vi "Mask Joysticks.vi"(6 "Operator POVs":i16[](array[numeric]), 7 "Driver Axes":dbl[](array[numeric])=[6.0, 0.0, 0.0, 1.0], 8 "Operator Buttons":bool[](array[boolean])=[FALSE, FALSE, FALSE, FALSE, FALSE, FALSE, FALSE, FALSE, FALSE, FALSE], 9 "Operator Axes":dbl[](array[numeric])=[6.0, 0.0, 0.0, 1.0], 10 "Driver POVs":i16[](array[numeric]), 11 "Driver Buttons":bool[](array[boolean])=[FALSE, FALSE, FALSE, FALSE, FALSE, FALSE, FALSE, FALSE, FALSE, FALSE]) -> (0 "Operator Buttons Out":bool[](array[boolean]), 1 "Operator Axes Out":dbl[](array[numeric])=[0.0, 0.0, 0.0, 1.0], 2 "Driver POVs Out":i16[](array[numeric]), 3 "Drive Buttons Out":bool[](array[boolean]), 4 "Operator POVs Out":i16[](array[numeric]), 5 "Drive Axes Out":dbl[](array[numeric])=[0.0, 0.0, 0.0, 1.0])   [LabVIEW 2018]
panel:
  in  "Operator Axes Mask":bool[](array[boolean])=[TRUE, TRUE, TRUE, TRUE, TRUE, TRUE, TRUE, TRUE, TRUE, TRUE]
  in  "Operator Buttons Mask":bool[](array[boolean])=[TRUE, TRUE, TRUE, TRUE, TRUE, TRUE, TRUE, TRUE, TRUE, TRUE]
  in  "D315":bool
  in  "D270":bool
  in  "D235":bool
  in  "D135":bool
  in  "D180":bool
  in  "D90":bool
  in  "D45":bool
  in  "D0/360":bool
  in  "Driver Buttons Mask":bool[](array[boolean])=[TRUE, TRUE, TRUE, TRUE, TRUE, TRUE, TRUE, TRUE, TRUE, TRUE]
  in  "Driver Axes Mask":bool[](array[boolean])=[TRUE, TRUE, TRUE, TRUE, TRUE, TRUE, TRUE, TRUE, TRUE, TRUE]
  # "POV Mask"
  # "POV Masking Not DOne"
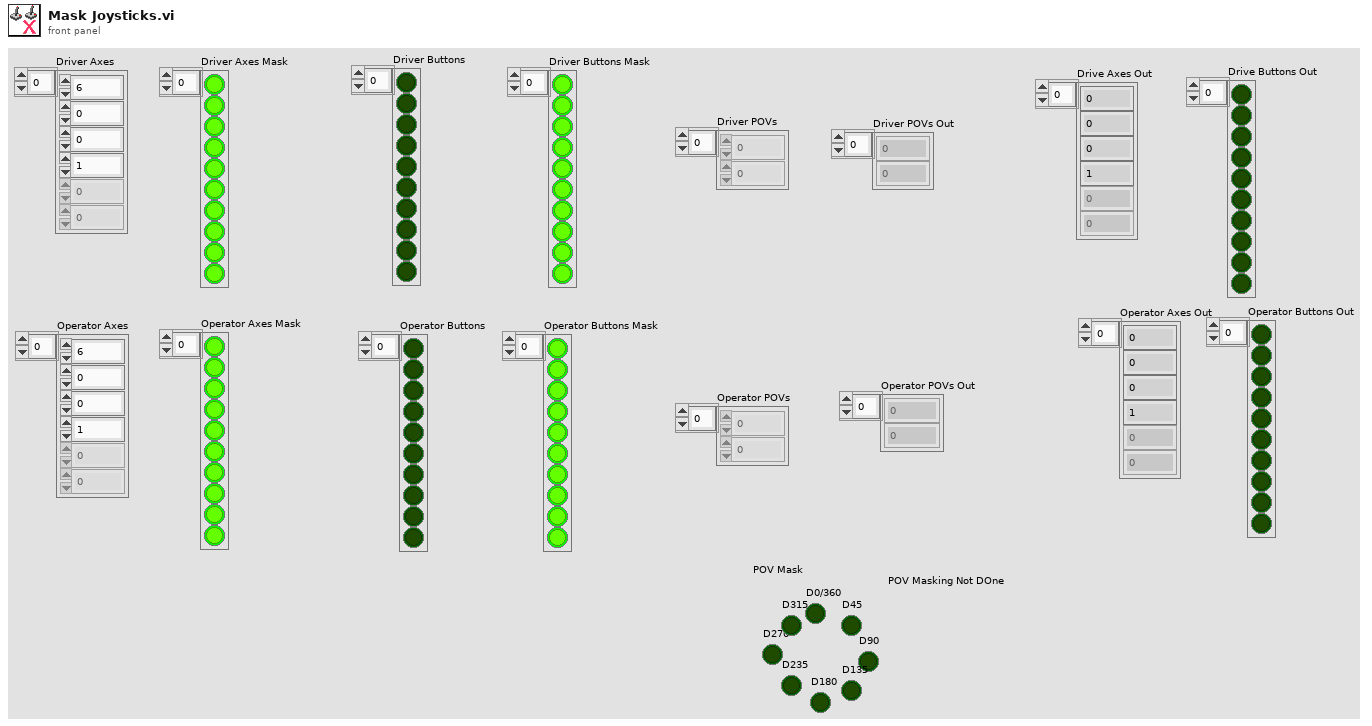
[diagram p1: front panel]
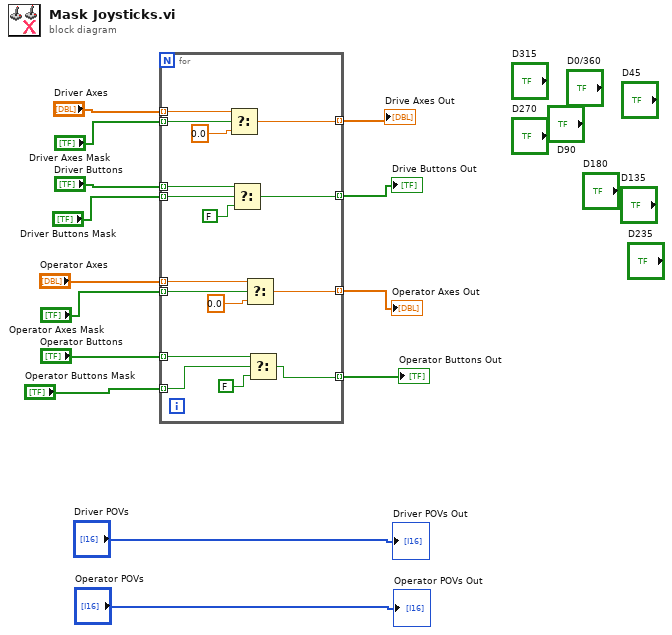
[diagram p0: block diagram]
diagram:
  n1 = for {
    tunnel: "Driver Axes Mask" -> [w30] mode=indexing
    tunnel: "Driver Axes" -> [w29] mode=indexing
    tunnel: "Driver Buttons Mask" -> [w27] mode=indexing
    tunnel: "Driver Buttons" -> [w26] mode=indexing
    tunnel: [w24] -> w9 mode=indexing
    tunnel: [w23] -> w8 mode=indexing
    tunnel: [w20] -> w7 mode=indexing
    tunnel: [w19] -> w6 mode=indexing
    tunnel: "Operator Axes" -> [w18] mode=indexing
    tunnel: "Operator Axes Mask" -> [w17] mode=indexing
    tunnel: "Operator Buttons" -> [w16] mode=indexing
    tunnel: "Operator Buttons Mask" -> [w15] mode=indexing
    n2 = Select(t=w29, s=w30, f=0.0) -> (s? t:f=w24:dbl)
    n3 = Select(t=w26, s=w27, f=FALSE) -> (s? t:f=w23:bool)
    n4 = Select(t=w18, s=w17, f=0.0) -> (s? t:f=w20:dbl)
    n5 = Select(t=w16, s=w15, f=FALSE) -> (s? t:f=w19:bool)
  }
  "Drive Axes Out" <- w9
  "Drive Buttons Out" <- w8
  "Operator Axes Out" <- w7
  "Operator Buttons Out" <- w6
  "Driver POVs Out" <- "Driver POVs"
  "Operator POVs Out" <- "Operator POVs"
